vi "ReadStream routeguide_RouteGuide_ListFeatures.vi"(8 "error in":errorcluster, 11 "Call ID in":T3) -> (0 "error out":errorcluster, 1 "Success":bool, 2 "Response Data":T1, 3 "Call ID":T3)   [LabVIEW 2019, in "route_guide_client.lvlib"]
uses:
  route_guide_client.lvlib
  <vilib>/gRPC/LabVIEW gRPC Library/Server API/typeDefs/grpcId.ctl
  RPC Messages/routeguide_Feature.ctl
  RPC Messages/routeguide_Point.ctl
  aea5dbbb-03a2-479b-ad95-94da4ee1cea9.vi
  <vilib>/gRPC/LabVIEW gRPC Library/Server API/Server/Get Server DLL Path.vi
  <vilib>/gRPC/LabVIEW gRPC Library/gprc-lvsupport-release.lvlib
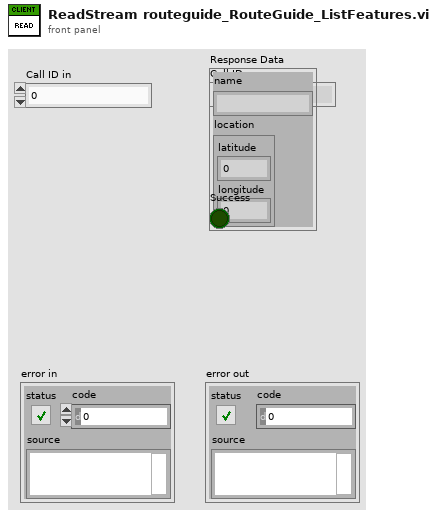
[diagram p1: front panel]
types:
  T1 = typedef "route_guide_client.lvlib/routeguide_Feature.ctl" = cluster{"name":string, "location":T2}
  T2 = typedef "route_guide_client.lvlib/routeguide_Point.ctl" = cluster{"latitude":i32, "longitude":i32}
  T3 = typedef "gprc-lvsupport-release.lvlib/grpcId.ctl" = u64
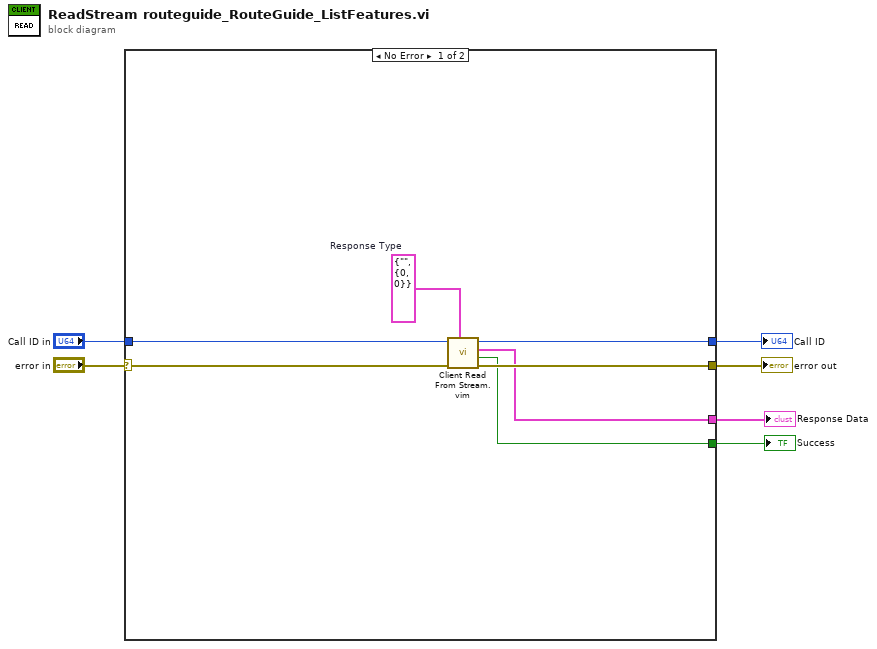
[diagram p0: block diagram]
diagram:
  n1 = case shown="No Error" "error in" {
    selector: "error in" -> [w13 w14]
    tunnel: [w12 w14] -> w5
    tunnel: "Call ID in" -> [w11 w15]
    tunnel: [w7 w15] -> w3
    tunnel: [w10 _] -> w2
    tunnel: [w8 _] -> w1
    frame No Error {
      w9 = T1 {"name"="", "location"={"latitude"=0, "longitude"=0}}  # Response Type
      n2 = call "Client Read From Stream.vim"("Response Type"=w9, "error in (no error)"=w13, "Call Id in"=w11) -> ("error out"=w12:errorcluster, "Success"=w8:bool, "Response Data"=w10:T1, "Call Id Out"=w7:u64)  [unwired: 5 in]
    }
    frame Error {
    }
  }
  "error out" <- w5
  "Call ID" <- w3
  "Response Data" <- w2
  "Success" <- w1
